vi "SimulateSignal.vi"(1 "Source":T1) -> (0 "Waveform Graph":dynamicdata(graph))   [LabVIEW 2014]
uses:
  sourceTypeDef.ctl
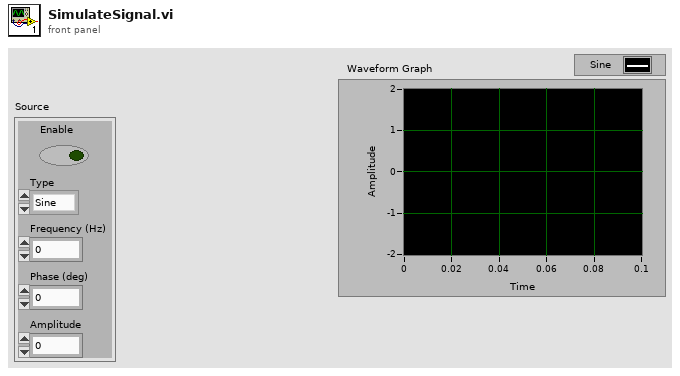
[diagram p1: front panel]
types:
  T1 = typedef "sourceTypeDef.ctl" = cluster{"Type":enum16{"Sine", "Square", "Triangle", "Noise"}, "Frequency (Hz)":dbl, "Phase (deg)":dbl, "Amplitude":dbl, "Enable":bool}
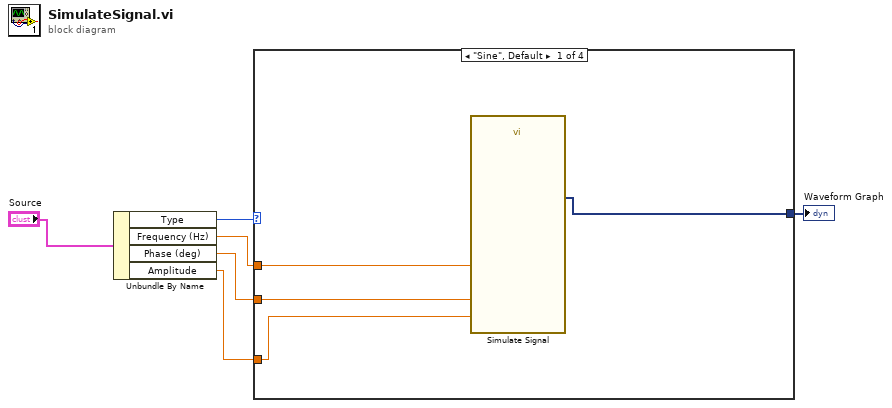
[diagram p0: block diagram]
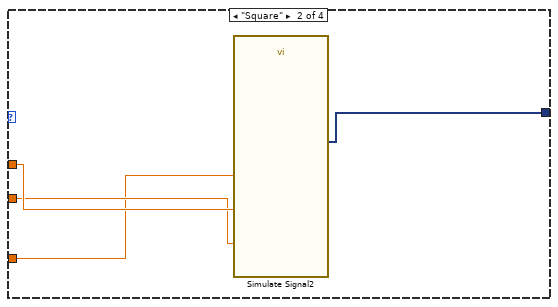
[diagram p2: hidden frame]
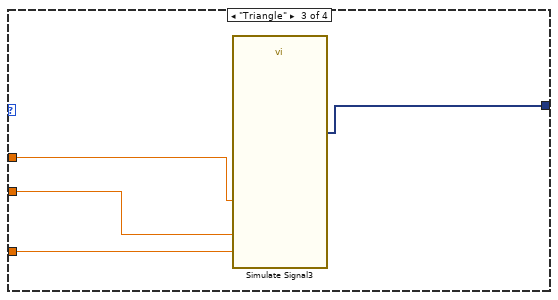
[diagram p3: hidden frame]
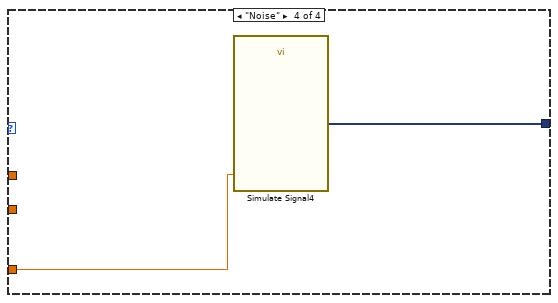
[diagram p4: hidden frame]
diagram:
  n1 = Unbundle By Name("Source") -> ("Type"=w4:enum16{"Sine", "Square", "Triangle", "Noise"}, "Frequency (Hz)"=w3:dbl, "Phase (deg)"=w2:dbl, "Amplitude"=w1:dbl)
  n2 = case shown="\"Sine\", Default" w4 {
    tunnel: w3 -> [w10 w14 w18 _]
    tunnel: w2 -> [w9 w13 w17 _]
    tunnel: [w8 w12 w16 w20] -> w6
    tunnel: w1 -> [w7 w11 w15 w19]
    frame "Sine", Default {
      n3 = call "Simulate Signal"("Frequency"=w10, "Amplitude"=w7, "Phase"=w9) -> ("Sine"=w8:dynamicdata)  [unwired: 11 in, 1 out]
    }
    frame "Square" {
      n4 = call "Simulate Signal2"("Frequency"=w14, "Amplitude"=w11, "Phase"=w13) -> ("Square"=w12:dynamicdata)  [unwired: 11 in, 1 out]
    }
    frame "Triangle" {
      n5 = call "Simulate Signal3"("Frequency"=w18, "Amplitude"=w15, "Phase"=w17) -> ("Triangle"=w16:dynamicdata)  [unwired: 11 in, 1 out]
    }
    frame "Noise" {
      n6 = call "Simulate Signal4"("Noise amplitude"=w19) -> ("DC with Uniform Noise"=w20:dynamicdata)  [unwired: 13 in, 1 out]
    }
  }
  "Waveform Graph" <- w6
